vi "apply channel changes.vi"(8 "error in":errorcluster, 9 "new channel":refnum<class "TBM channel.lvclass">, 10 "old channel":refnum<class "TBM channel.lvclass">, 11 "Scaling configuration in":refnum<class "Scaling configuration.lvclass">) -> (0 "error out":errorcluster, 3 "Scaling configuration out":refnum<class "Scaling configuration.lvclass">)   [LabVIEW 2013, in "Scaling configuration.lvclass"]
uses:
  Scaling configuration.lvclass
  <vilib>/NI/Tag Bus Module Framework/channel/TBM channel.lvclass
  <vilib>/NI/Tag Bus/tag/tag descriptor.lvclass
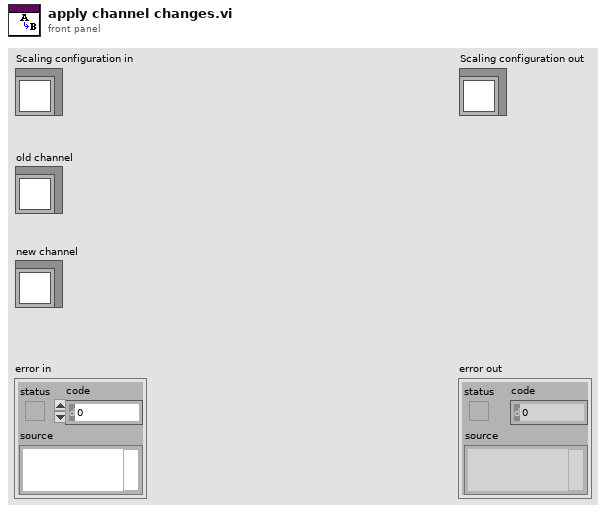
[diagram p1: front panel]
types:
  T1 = typedef "Scaling configuration.lvclass/scale data types.ctl" = enum16{"Double", "Single", "I64", "I32", "I16", "I8", "U64", "U32", "U16", "U8"}
  T2 = cluster{"input channel":refnum<class "TBM channel.lvclass">, "output channel":refnum<class "TBM channel.lvclass">, "input data type":T1, "output data type":T1}[][]
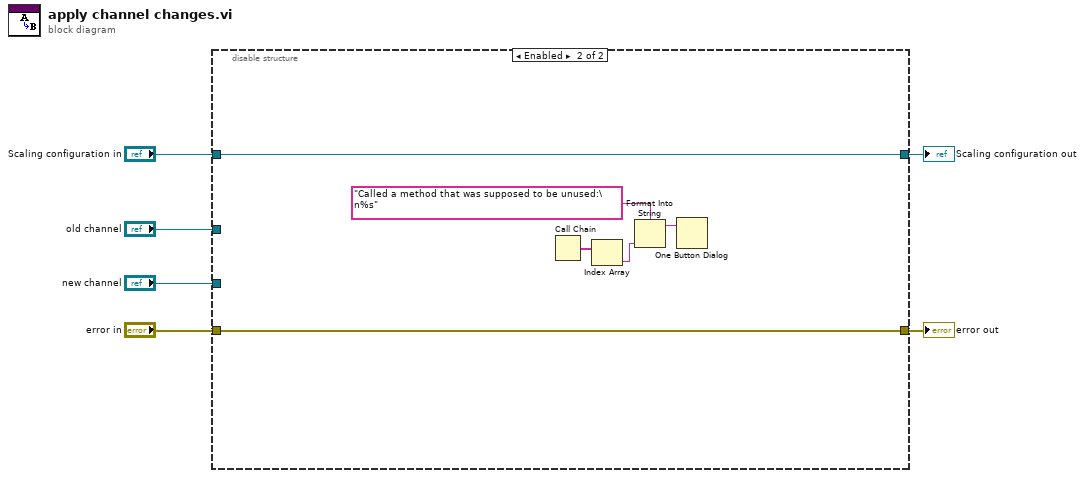
[diagram p0: block diagram]
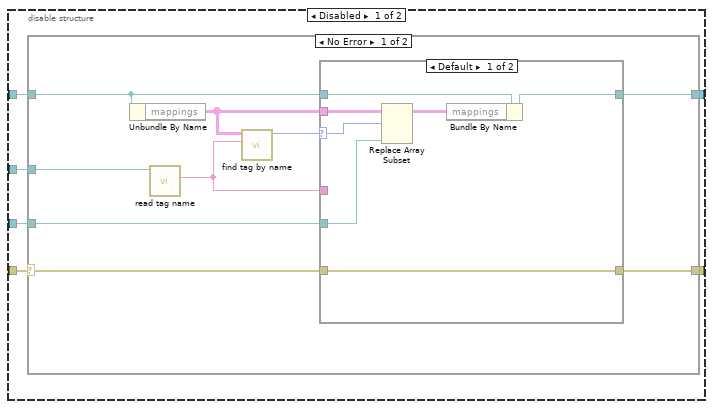
[diagram p2: hidden frame]
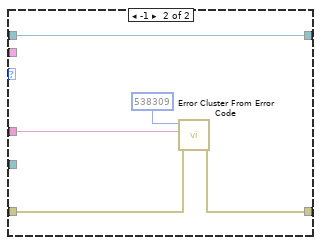
[diagram p3: hidden frame]
diagram:
  n1 = disable-structure shown="Enabled" {
    disable-tunnel: "error in" -> [w12 w41]
    disable-tunnel: [w11 w41] -> w5
    disable-tunnel: "Scaling configuration in" -> [w10 w40]
    disable-tunnel: [w9 w40] -> w3
    disable-tunnel: "old channel" -> [w8 _]
    disable-tunnel: "new channel" -> [w7 _]
    frame Disabled {
      n2 = case shown="No Error" w12 {
        selector: w12 -> [w16 w35]
        tunnel: [w15 w35] -> w11
        tunnel: [w19 w34] -> w9
        tunnel: w10 -> [w20 w34]
        tunnel: w8 -> [w21 _]
        tunnel: w7 -> [w17 _]
        frame No Error {
          n3 = Unbundle By Name(w20) -> ("mappings"=w18:T2)
          n4 = call <vilib>:"read tag name.vi"("system tag in"=w21) -> ("name"=w13:string)  [unwired: 8 in, 2 out]
          n5 = call <vilib>:"find tag by name.vi"("name"=w13, "tags in"=w18) -> ("index"=w14:i32)  [unwired: 9 in]
          n6 = case shown="Default" w14 {
            selector: w14 -> [w26 _]
            tunnel: w20 -> [w28 w33]
            tunnel: [w25 w33] -> w19
            tunnel: w18 -> [w27 _]
            tunnel: w17 -> [w23 _]
            tunnel: w13 -> [_ w31]
            tunnel: w16 -> [w22 w30]
            tunnel: [w22 w29] -> w15
            frame Default {
              n7 = Replace Array Subset(array=w27, new element=w23, index (row)=w26) -> (w24:T2)  [unwired: 1 in]
              n8 = Bundle By Name(cluster=w28, "mappings"=w24) -> (w25:refnum<class "Scaling configuration.lvclass">)
            }
            frame -1 {
              n9 = call <vilib>:"Error Cluster From Error Code.vi"("error in (no error)"=w30, "error message (\"\")"=w31, "error code (0)"=538309) -> ("error out"=w29:errorcluster)  [unwired: 6 in]
            }
          }
        }
        frame Error {
        }
      }
    }
    frame Enabled {
      n10 = Call Chain() -> (call chain=w39:string[])
      n11 = Index Array(array=w39) -> (element=w38:string)  [unwired: 1 in]
      n12 = Format Into String(format string="Called a method that was supposed to be unused:\n%s", w38) -> (resulting string=w36:string)  [unwired: 2 in, 1 out]
      n13 = One Button Dialog(message=w36) -> ()  [unwired: 1 in, 1 out]
    }
  }
  "error out" <- w5
  "Scaling configuration out" <- w3
